vi "PicoScope5000aGetBlock.vi"(0 "error in":errorcluster, 1 "stop IsReady":bool, 2 "handle in":i16, 3 "Acquisition Settings":T3 {"Down Sample Ratio" min=1 step=1; "Down-Sample Mode" items=["None", "Aggregate", "Decimate", "Average"]}, 5 "enabled array":i16[](array[numeric])) -> (4 "overflow":i16, 6 "error out":errorcluster, 7 "handle out":i16, 8 "noOfSamples":u32, 9 "Buffers (Max or non-aggregated)":T1, 10 "Min Buffers":T2)   [LabVIEW 2009]
doc: "This VI collects a block of data from the oscilloscope. This can be called in a loop in order to continually collect blocks of data. The oscilloscope should first be set up by using PicoScope3000aSettings.vi. The VI outputs data arrays in two clusters (max and min). If not using aggregation, 'Min Buffers' is not used."
uses:
  ps5000a.dll
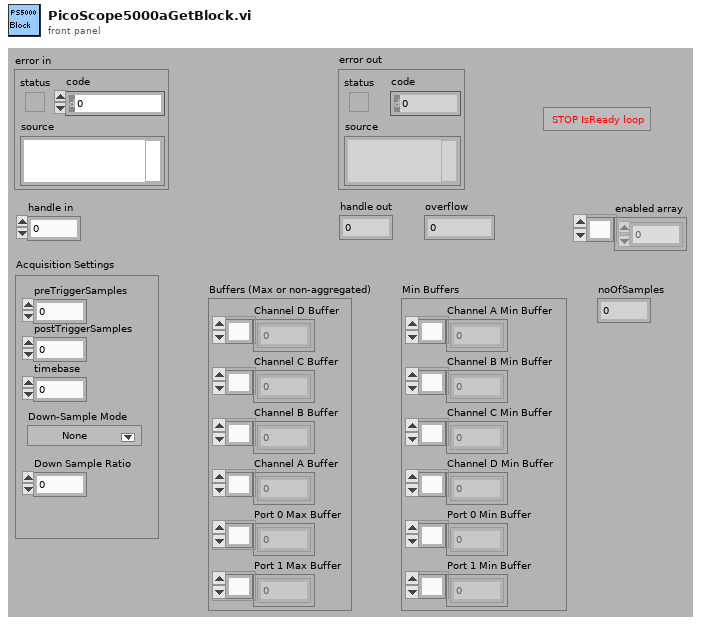
[diagram p1: front panel]
types:
  T1 = cluster{"Channel D Buffer":i16[], "Channel C Buffer":i16[], "Channel B Buffer":i16[], "Channel A Buffer":i16[], "Port 0 Max Buffer":i32[], "Port 1 Max Buffer":i32[]}
  T2 = cluster{"Channel A Min Buffer":i16[], "Channel B Min Buffer":i16[], "Channel C Min Buffer":i16[], "Channel D Min Buffer":i16[], "Port 0 Min Buffer":i32[], "Port 1 Min Buffer":i32[]}
  T3 = cluster{"preTriggerSamples":i32, "postTriggerSamples":i32, "timebase":u32, "Down-Sample Mode":u32, "Down Sample Ratio":u32}
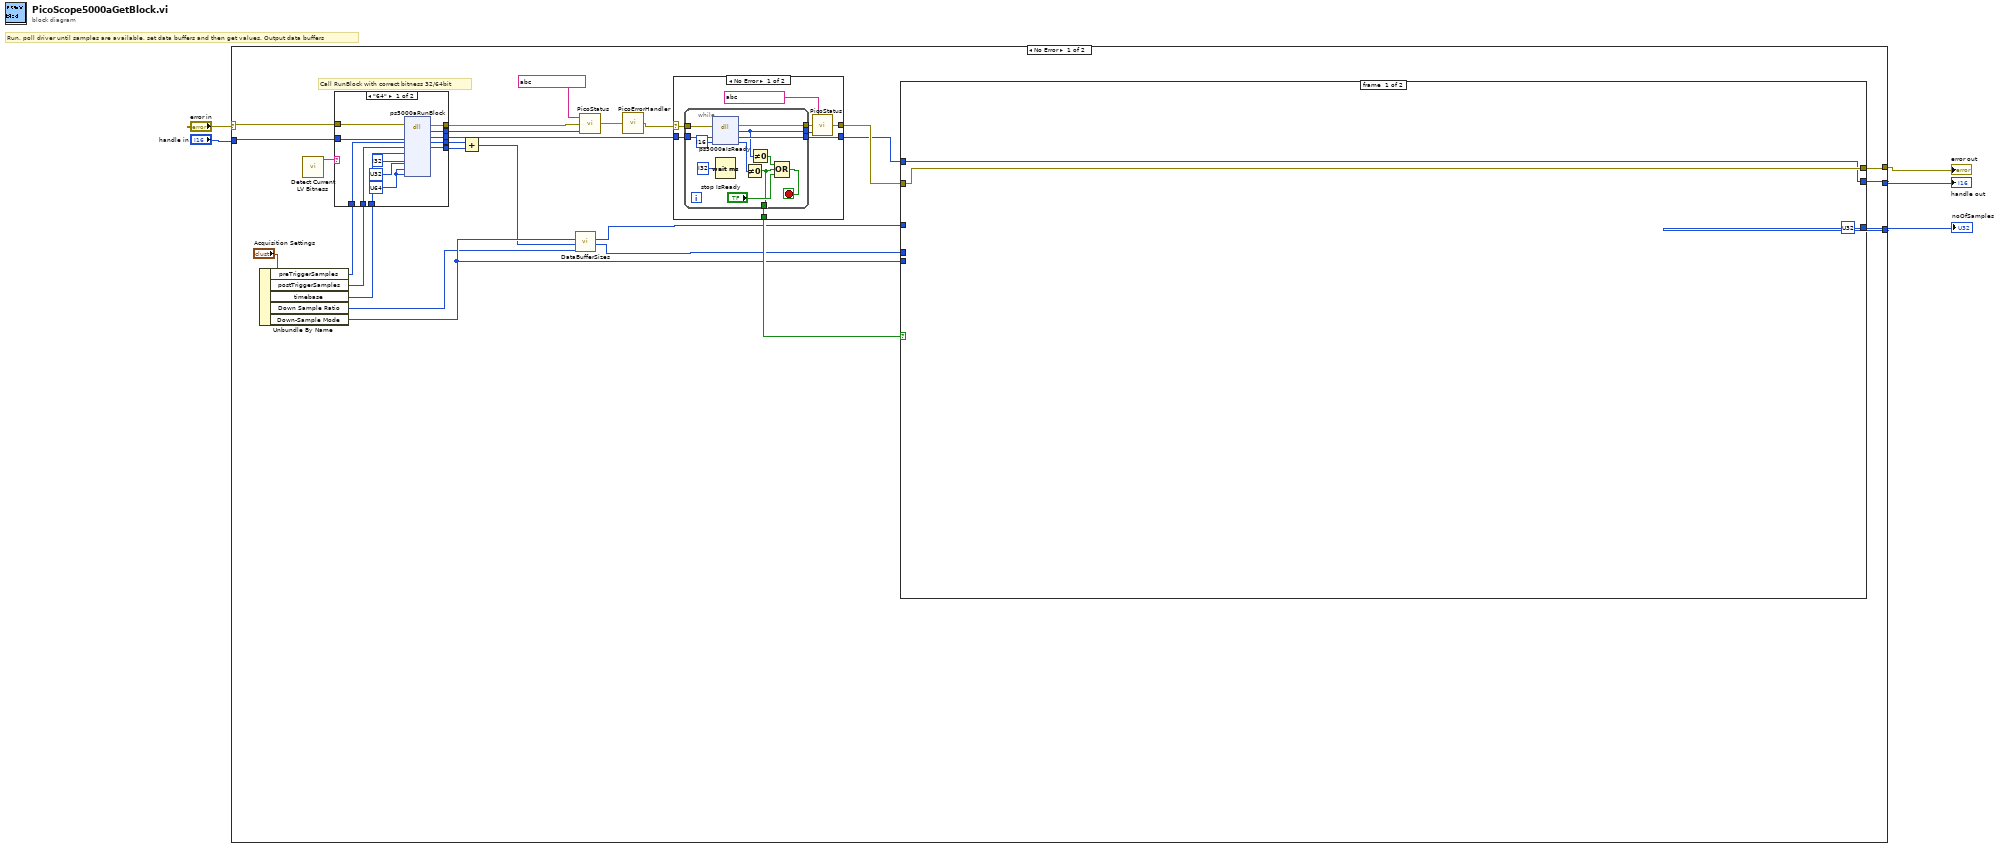
[diagram p0: block diagram]
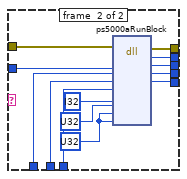
[diagram p2: hidden frame]
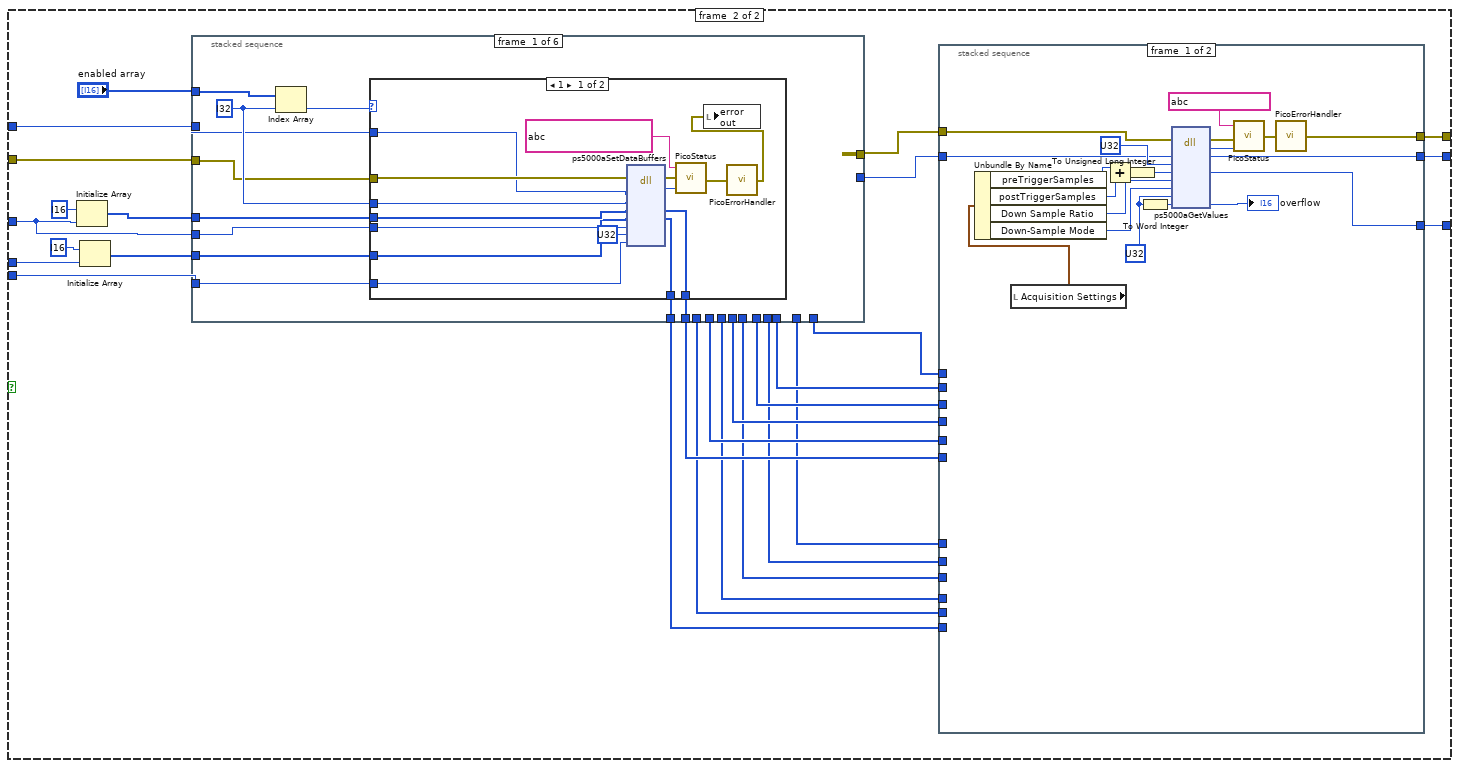
[diagram p3: hidden frame]
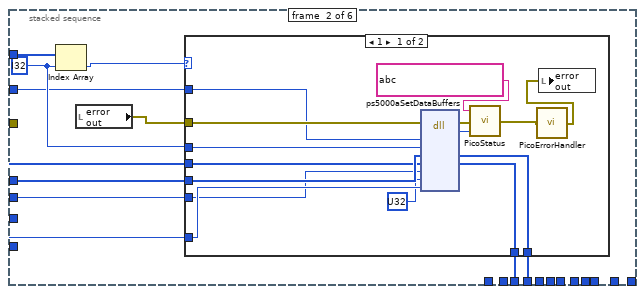
[diagram p5: hidden frame]
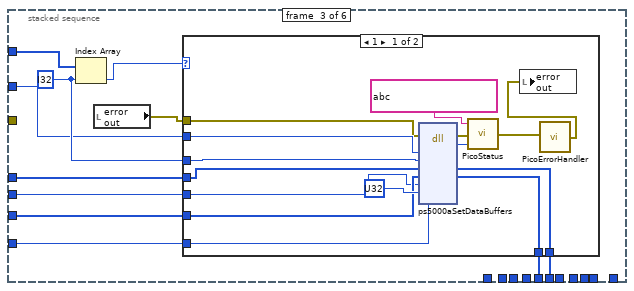
[diagram p7: hidden frame]
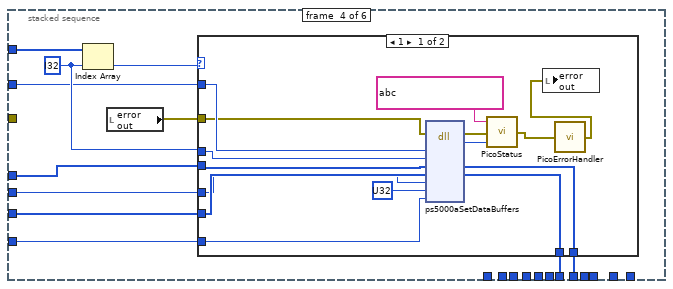
[diagram p9: hidden frame]
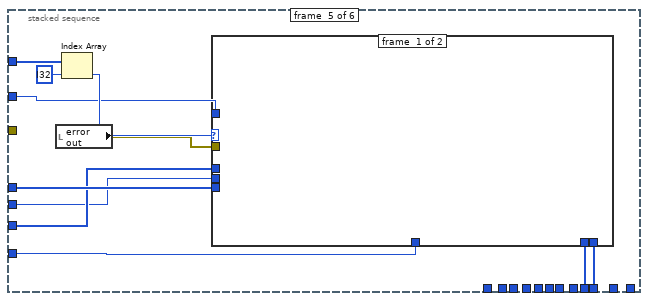
[diagram p11: hidden frame]
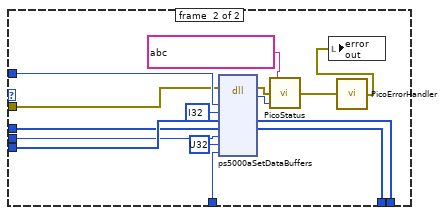
[diagram p12: hidden frame]
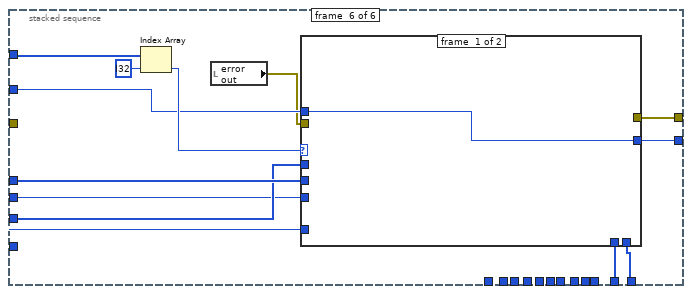
[diagram p13: hidden frame]
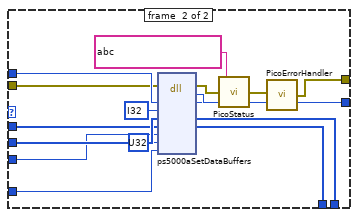
[diagram p14: hidden frame]
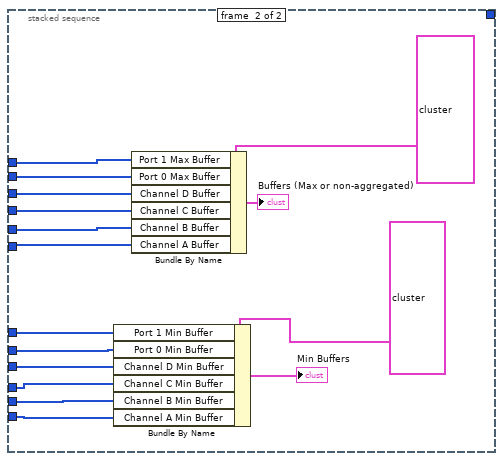
[diagram p15: hidden frame]
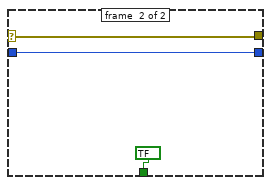
[diagram p16: hidden frame]
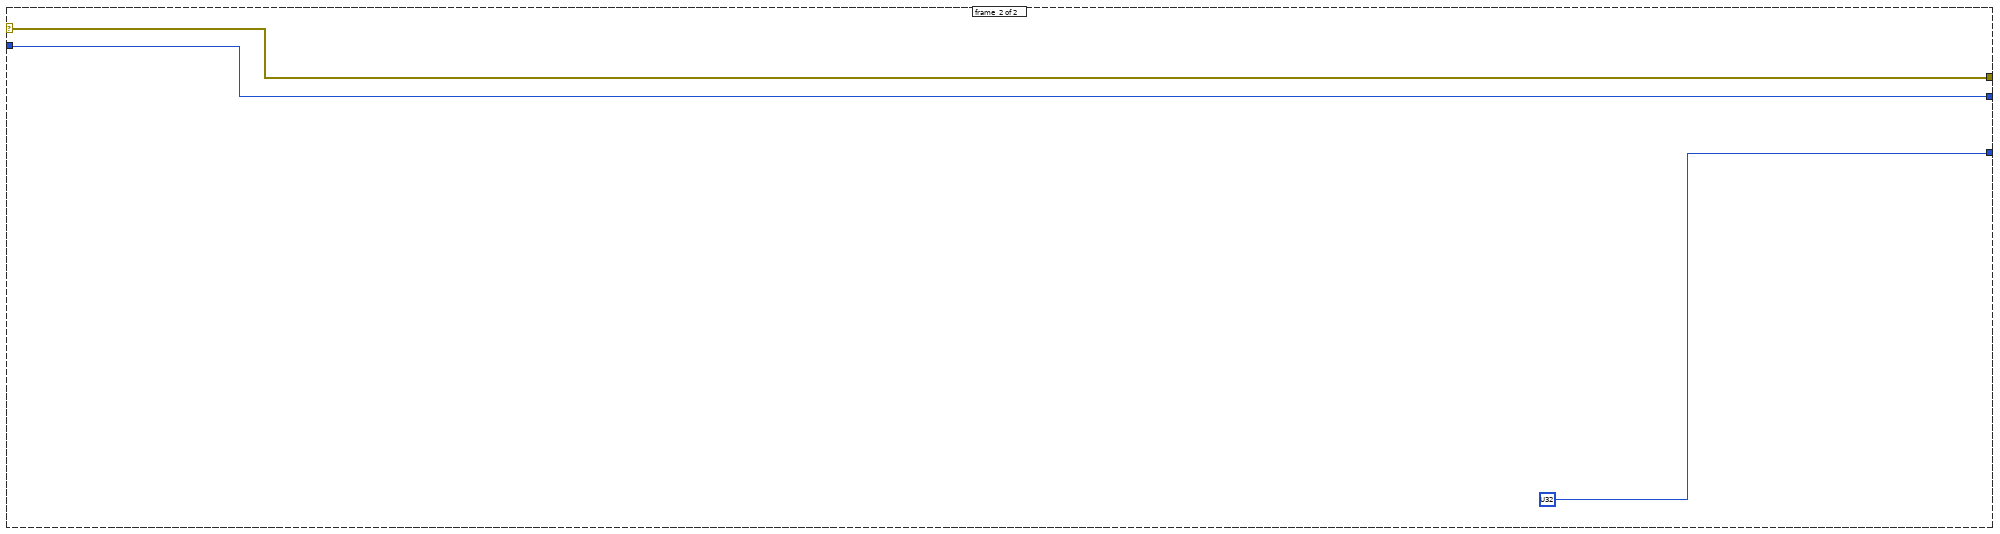
[diagram p17: hidden frame]
diagram:
  # "Run, poll driver until samples are available, set data buffers and then get values. Output data buffers"
  n1 = case shown="No Error" "error in" {
    selector: "error in" -> [w24 w309]
    tunnel: [w25 w309] -> w5
    tunnel: "handle in" -> [w23 w308]
    tunnel: [w22 w308] -> w4
    tunnel: [w17 u32 ? ("noOfSamples")] -> w1
    frame #0 {
      # "Call RunBlock with correct bitness 32/64bit"
      n2 = Unbundle By Name("Acquisition Settings") -> ("preTriggerSamples"=w21:i32, "postTriggerSamples"=w20:i32, "timebase"=w19:u32, "Down Sample Ratio"=w8:u32, "Down-Sample Mode"=w10:u32)
      n3 = call "Detect Current LV Bitness.vi"() -> ("bitness"=w11:string)  [unwired: 11 in]
      n4 = case shown="\"64\"" w11 {
        tunnel: [w44 w57] -> w31
        tunnel: [w43 w56] -> w30
        tunnel: [w42 w55] -> w28
        tunnel: [w41 w54] -> w27
        tunnel: w24 -> [w40 w53]
        tunnel: w23 -> [w39 w52]
        tunnel: w21 -> [w38 w51]
        tunnel: w20 -> [w37 w50]
        tunnel: w19 -> [w36 w49]
        tunnel: [w35 w48] -> w15
        frame #0 {
          w32 = u64 ? ("pParameter")
          n5 = dll-call lib="ps5000a.dll" fn="ps5000aRunBlock" ("ps3000.dll:_ps3000_open_unit@0")(error in=w40, "handle"=w39, "preTriggerSamples"=w38, "postTriggerSamples"=w37, "timebase"=w36, "timeindisposed"=i32 ? ("pParameter"), "segmentIndex"=u32 ? ("pParameter"), "lpReady"=w32, "pParameter"=w32) -> (error out=w41:errorcluster, "PICO_STATUS"=w42:u32, "handle"=w35:i16, "preTriggerSamples"=w44:i32, "postTriggerSamples"=w43:i32)  [unwired: 7 in, 1 out]
        }
        frame #1 {
          w45 = u32 ? ("pParameter")
          n6 = dll-call lib="ps5000a.dll" fn="ps5000aRunBlock" ("ps3000.dll:_ps3000_open_unit@0")(error in=w53, "handle"=w52, "preTriggerSamples"=w51, "postTriggerSamples"=w50, "timebase"=w49, "timeindisposed"=i32 ? ("pParameter"), "segmentIndex"=u32 ? ("pParameter"), "lpReady"=w45, "pParameter"=w45) -> (error out=w54:errorcluster, "PICO_STATUS"=w55:u32, "handle"=w48:i16, "preTriggerSamples"=w57:i32, "postTriggerSamples"=w56:i32)  [unwired: 7 in, 1 out]
        }
      }
      n7 = Add(x=w31, y=w30) -> (x+y=w9:i32)
      n8 = call "DataBufferSizes.vi"("Down Sample Ratio"=w8, "Number of Samples"=w9, "Down-Sample Mode"=w10) -> ("min Buffer Size"=w6:i32, "Max Buffer Size"=w7:i32)  [unwired: 7 in]
      n9 = call "PicoStatus.vi"("PICO STATUS"=w28, "error in"=w27, "source"=string ?) -> ("error out"=w18:errorcluster)
      n10 = call "PicoErrorHandler.vi"("error in"=w18) -> ("error out"=w16:errorcluster)
      n11 = case shown="No Error" w16 {
        selector: w16 -> [w289 w305]
        tunnel: w15 -> [w291 w306]
        tunnel: [w290 w306] -> w13
        tunnel: [w288 w305] -> w14
        tunnel: [w284 bool ?] -> w12
        frame #0 {
          n12 = while {
            tunnel: [w303] -> w290
            tunnel: w291 -> [w302]
            tunnel: [w300] -> w286
            tunnel: w289 -> [w299]
            tunnel: [w298] -> w287
            tunnel: [w292] -> w284
            stop <- w295 stop-if-true
            n13 = dll-call lib="ps5000a.dll" fn="ps5000aIsReady" ("ps3000.dll:_ps3000_open_unit@0")(error in=w299, "handle"=w302, "ready"=i16 ?) -> (error out=w298:errorcluster, "PICO_STATUS"=w300:u32, "handle"=w303:i16, "ready"=w301:i16)  [unwired: 2 in, 1 out]
            n14 = Wait (ms)(milliseconds to wait=i32 ?) -> ()  [unwired: 1 out]
            n15 = Not Equal To 0?(x=w301) -> (x != 0?=w292:bool)
            n16 = Not Equal To 0?(x=w300) -> (x != 0?=w294:bool)
            n17 = Compound Arithmetic op=OR(w294, w292, "stop IsReady") -> (w295:bool)
          }
          n18 = call "PicoStatus.vi"("PICO STATUS"=w286, "error in"=w287, "source"=string ?) -> ("error out"=w288:errorcluster)
        }
        frame #1 {
        }
      }
      n19 = case shown="True" w12 {
        tunnel: [w60 w87] -> w25
        tunnel: [w59 w86] -> w22
        tunnel: [u32 ? ("noOfSamples") w85] -> w17
        tunnel: w14 -> [w60 w81]
        tunnel: w13 -> [w59 w80]
        tunnel: w7 -> [_ w61]
        tunnel: w6 -> [_ w63]
        tunnel: w10 -> [_ w62]
        frame #0 {
        }
        frame #1 {
          n20 = Initialize Array(i16 ? ("element"), w61) -> (w79:i16[])
          n21 = Initialize Array(i16 ? ("element"), w63) -> (w78:i16[])
          n22 = stacked-sequence {
            tunnel: "enabled array" -> [w97 w122 w149 w174 w202 w230]
            tunnel: w81 -> [w95 _ _ _ _ _]
            tunnel: w80 -> [w94 w121 w147 w173 w199 w227]
            tunnel: w79 -> [w93 w120 w146 w172 w198 w226]
            tunnel: w78 -> [w92 w119 w145 w171 w197 w225]
            tunnel: w61 -> [w91 w117 w144 w170 w196 w224]
            tunnel: w62 -> [w90 w118 w143 w169 w195 w223]
            tunnel: [w89 _ _ _ _ _] -> w77
            tunnel: [w88 _ _ _ _ _] -> w76
            tunnel: [_ w116 _ _ _ _] -> w75
            tunnel: [_ w115 _ _ _ _] -> w74
            tunnel: [_ _ w142 _ _ _] -> w73
            tunnel: [_ _ w141 _ _ _] -> w72
            tunnel: [_ _ _ w168 _ _] -> w71
            tunnel: [_ _ _ w167 _ _] -> w70
            tunnel: [_ _ _ _ w194 _] -> w69
            tunnel: [_ _ _ _ w193 _] -> w68
            tunnel: [_ _ _ _ _ w222] -> w67
            tunnel: [_ _ _ _ _ w221] -> w66
            tunnel: [_ _ _ _ _ w220] -> w65
            tunnel: [_ _ _ _ _ w218] -> w64
            frame #0 {
              w98 = i32 ? ("dimension size")
              n23 = Index Array(array=w97, index=w98) -> (element=w96:i16)
              n24 = case shown="1" w96 {
                tunnel: w98 -> [w107 _]
                tunnel: w95 -> [w112 _]
                tunnel: w94 -> [w109 _]
                tunnel: w93 -> [w106 _]
                tunnel: w92 -> [w105 _]
                tunnel: w91 -> [w104 _]
                tunnel: w90 -> [w103 _]
                tunnel: [w100 _] -> w89
                tunnel: [w99 _] -> w88
                frame #0 {
                  n25 = dll-call lib="ps5000a.dll" fn="ps5000aSetDataBuffers" ("ps3000.dll:_ps3000_open_unit@0")(error in=w112, "handle"=w109, "channel"=w107, "bufferMax"=w106, "bufferMin"=w105, "bufferLth"=w104, "segmentIndex"=u32 ?, "mode"=w103) -> (error out=w111:errorcluster, "PICO_STATUS"=w110:u32, "bufferMax"=w99:i16[], "bufferMin"=w100:i16[])  [unwired: 7 in, 1 out]
                  n26 = call "PicoStatus.vi"("PICO STATUS"=w110, "error in"=w111, "source"=string ?) -> ("error out"=w113:errorcluster)
                  n27 = call "PicoErrorHandler.vi"("error in"=w113) -> ("error out"=w101:errorcluster)
                  n28 = local write "error out"(w101) -> ()
                }
                frame #1 {
                }
              }
            }
            frame #1 {
              w124 = i32 ? ("dimension size")
              n29 = Index Array(array=w122, index=w124) -> (element=w123:i16)
              n30 = local read "error out"() -> (w114:errorcluster)
              n31 = case shown="1" w123 {
                tunnel: w124 -> [w134 _]
                tunnel: w114 -> [w133 _]
                tunnel: w121 -> [w132 _]
                tunnel: w120 -> [w131 _]
                tunnel: w119 -> [w130 _]
                tunnel: w118 -> [w129 _]
                tunnel: w117 -> [w127 _]
                tunnel: [w126 _] -> w116
                tunnel: [w125 _] -> w115
                frame #0 {
                  n32 = dll-call lib="ps5000a.dll" fn="ps5000aSetDataBuffers" ("ps3000.dll:_ps3000_open_unit@0")(error in=w133, "handle"=w132, "channel"=w134, "bufferMax"=w131, "bufferMin"=w130, "bufferLth"=w127, "segmentIndex"=u32 ?, "mode"=w129) -> (error out=w138:errorcluster, "PICO_STATUS"=w139:u32, "bufferMax"=w125:i16[], "bufferMin"=w126:i16[])  [unwired: 7 in, 1 out]
                  n33 = call "PicoStatus.vi"("PICO STATUS"=w139, "error in"=w138, "source"=string ?) -> ("error out"=w135:errorcluster)
                  n34 = call "PicoErrorHandler.vi"("error in"=w135) -> ("error out"=w136:errorcluster)
                  n35 = local write "error out"(w136) -> ()
                }
                frame #1 {
                }
              }
            }
            frame #2 {
              w150 = i32 ? ("dimension size")
              n36 = Index Array(array=w149, index=w150) -> (element=w148:i16)
              n37 = local read "error out"() -> (w140:errorcluster)
              n38 = case shown="1" w148 {
                tunnel: w150 -> [w161 _]
                tunnel: w147 -> [w160 _]
                tunnel: w146 -> [w159 _]
                tunnel: w145 -> [w158 _]
                tunnel: w144 -> [w157 _]
                tunnel: w143 -> [w156 _]
                tunnel: [w153 _] -> w142
                tunnel: [w152 _] -> w141
                tunnel: w140 -> [w151 _]
                frame #0 {
                  n39 = dll-call lib="ps5000a.dll" fn="ps5000aSetDataBuffers" ("ps3000.dll:_ps3000_open_unit@0")(error in=w151, "handle"=w160, "channel"=w161, "bufferMax"=w159, "bufferMin"=w158, "bufferLth"=w157, "segmentIndex"=u32 ?, "mode"=w156) -> (error out=w164:errorcluster, "PICO_STATUS"=w165:u32, "bufferMax"=w152:i16[], "bufferMin"=w153:i16[])  [unwired: 7 in, 1 out]
                  n40 = call "PicoStatus.vi"("PICO STATUS"=w165, "error in"=w164, "source"=string ?) -> ("error out"=w155:errorcluster)
                  n41 = call "PicoErrorHandler.vi"("error in"=w155) -> ("error out"=w154:errorcluster)
                  n42 = local write "error out"(w154) -> ()
                }
                frame #1 {
                }
              }
            }
            frame #3 {
              w176 = i32 ? ("dimension size")
              n43 = Index Array(array=w174, index=w176) -> (element=w175:i16)
              n44 = local read "error out"() -> (w166:errorcluster)
              n45 = case shown="1" w175 {
                tunnel: w176 -> [w187 _]
                tunnel: w173 -> [w186 _]
                tunnel: w166 -> [w185 _]
                tunnel: w172 -> [w184 _]
                tunnel: w171 -> [w183 _]
                tunnel: w170 -> [w182 _]
                tunnel: w169 -> [w181 _]
                tunnel: [w178 _] -> w168
                tunnel: [w177 _] -> w167
                frame #0 {
                  n46 = dll-call lib="ps5000a.dll" fn="ps5000aSetDataBuffers" ("ps3000.dll:_ps3000_open_unit@0")(error in=w185, "handle"=w186, "channel"=w187, "bufferMax"=w184, "bufferMin"=w183, "bufferLth"=w182, "segmentIndex"=u32 ?, "mode"=w181) -> (error out=w190:errorcluster, "PICO_STATUS"=w191:u32, "bufferMax"=w177:i16[], "bufferMin"=w178:i16[])  [unwired: 7 in, 1 out]
                  n47 = call "PicoStatus.vi"("PICO STATUS"=w191, "error in"=w190, "source"=string ?) -> ("error out"=w180:errorcluster)
                  n48 = call "PicoErrorHandler.vi"("error in"=w180) -> ("error out"=w179:errorcluster)
                  n49 = local write "error out"(w179) -> ()
                }
                frame #1 {
                }
              }
            }
            frame #4 {
              n50 = local read "error out"() -> (w192:errorcluster)
              n51 = Index Array(array=w202, index=i32 ?) -> (element=w200:i16)
              n52 = case shown="1" w200 {
                tunnel: w199 -> [_ w211]
                tunnel: w192 -> [_ w210]
                tunnel: w198 -> [_ w209]
                tunnel: w197 -> [_ w208]
                tunnel: w196 -> [_ w207]
                tunnel: w195 -> [_ w205]
                tunnel: [_ w204] -> w194
                tunnel: [_ w203] -> w193
                frame #0 {
                }
                frame #1 {
                  n53 = dll-call lib="ps5000a.dll" fn="ps5000aSetDataBuffers"(error in=w210, "handle"=w211, "channel"=i32 ?, "bufferMax"=w209, "bufferMin"=w208, "bufferLth"=w207, "segmentIndex"=u32 ?, "mode"=w205) -> (error out=w216:errorcluster, "PICO_STATUS"=w217:u32, "bufferMax"=w203:i16[], "bufferMin"=w204:i16[])  [unwired: 7 in, 1 out]
                  n54 = call "PicoStatus.vi"("PICO STATUS"=w217, "error in"=w216, "source"=string ?) -> ("error out"=w213:errorcluster)
                  n55 = call "PicoErrorHandler.vi"("error in"=w213) -> ("error out"=w212:errorcluster)
                  n56 = local write "error out"(w212) -> ()
                }
              }
            }
            frame #5 {
              n57 = Index Array(array=w230, index=i32 ?) -> (element=w229:i16)
              n58 = local read "error out"() -> (w219:errorcluster)
              n59 = case shown="1" w229 {
                tunnel: w227 -> [w231 w244]
                tunnel: w219 -> [_ w243]
                tunnel: w226 -> [_ w242]
                tunnel: w225 -> [_ w241]
                tunnel: w224 -> [_ w240]
                tunnel: w223 -> [_ w238]
                tunnel: [_ w236] -> w222
                tunnel: [_ w235] -> w221
                tunnel: [_ w234] -> w220
                tunnel: [w231 w232] -> w218
                frame #0 {
                }
                frame #1 {
                  n60 = dll-call lib="ps5000a.dll" fn="ps5000aSetDataBuffers" ("ps3000.dll:_ps3000_open_unit@0")(error in=w243, "handle"=w244, "channel"=i32 ?, "bufferMax"=w242, "bufferMin"=w241, "bufferLth"=w240, "segmentIndex"=u32 ?, "mode"=w238) -> (error out=w247:errorcluster, "PICO_STATUS"=w233:u32, "handle"=w232:i16, "bufferMax"=w235:i16[], "bufferMin"=w236:i16[])  [unwired: 6 in, 1 out]
                  n61 = call "PicoStatus.vi"("PICO STATUS"=w233, "error in"=w247, "source"=string ?) -> ("error out"=w237:errorcluster)
                  n62 = call "PicoErrorHandler.vi"("error in"=w237) -> ("error out"=w234:errorcluster)
                }
              }
            }
          }
          n63 = stacked-sequence {
            tunnel: [w261 _] -> w87
            tunnel: [w260 _] -> w86
            tunnel: [w250 _] -> w85
            tunnel: w77 -> [_ w279]
            tunnel: w76 -> [_ w278]
            tunnel: w75 -> [_ w277]
            tunnel: w74 -> [_ w276]
            tunnel: w73 -> [_ w274]
            tunnel: w72 -> [_ w275]
            tunnel: w71 -> [_ w273]
            tunnel: w70 -> [_ w272]
            tunnel: w69 -> [_ w271]
            tunnel: w68 -> [_ w270]
            tunnel: w67 -> [_ w269]
            tunnel: w66 -> [_ w268]
            tunnel: w65 -> [w249 _]
            tunnel: w64 -> [w248 _]
            frame #0 {
              w266 = u32 ? ("overflow")
              n64 = local read "Acquisition Settings"() -> (w258:T3)
              n65 = Unbundle By Name(w258) -> ("preTriggerSamples"=w255:i32, "postTriggerSamples"=w256:i32, "Down Sample Ratio"=w257:u32, "Down-Sample Mode"=w253:u32)
              n66 = Add(x=w255, y=w256) -> (x+y=w254:i32)
              n67 = To Unsigned Long Integer(number=w254) -> (unsigned 32bit integer=w252:u32)
              n68 = To Word Integer(number=w266) -> (16bit integer=w251:i16)
              n69 = dll-call lib="ps5000a.dll" fn="ps5000aGetValues" ("ps3000.dll:_ps3000_open_unit@0")(error in=w249, "handle"=w248, "startIndex"=u32 ?, "noOfSamples"=w252, "downSampleRatio"=w257, "downSampleRatioMode"=w253, "segmentIndex"=w266, "overflow"=w251) -> (error out=w264:errorcluster, "PICO_STATUS"=w265:u32, "handle"=w260:i16, "noOfSamples"=w250:u32, "overflow"=→"overflow":i16)  [unwired: 6 in, 1 out]
              n70 = call "PicoStatus.vi"("PICO STATUS"=w265, "error in"=w264, "source"=string ?) -> ("error out"=w262:errorcluster)
              n71 = call "PicoErrorHandler.vi"("error in"=w262) -> ("error out"=w261:errorcluster)
            }
            frame #1 {
              n72 = Bundle By Name(cluster=T2 ? ("Min Buffers"), "Port 1 Min Buffer"=w269, "Port 0 Min Buffer"=w271, "Channel D Min Buffer"=w273, "Channel C Min Buffer"=w274, "Channel B Min Buffer"=w277, "Channel A Min Buffer"=w279) -> (→"Min Buffers":T2)
              n73 = Bundle By Name(cluster=T1 ? ("Buffers (Max or non-aggregated)"), "Port 1 Max Buffer"=w268, "Port 0 Max Buffer"=w270, "Channel D Buffer"=w272, "Channel C Buffer"=w275, "Channel B Buffer"=w276, "Channel A Buffer"=w278) -> (→"Buffers (Max or non-aggregated)":T1)
            }
          }
        }
      }
    }
    frame #1 {
    }
  }
  "error out" <- w5
  "handle out" <- w4
  "noOfSamples" <- w1
